vi "MotorParam_mm_to_ct.vi"(10 "Motor Parameters (Natural Units)":T1={"velocity mm/s"=[10.0, 10.0, 10.0, 20.0], "accel mm/s^2"=[50.0, 50.0, 50.0, 200.0]}, 11 "Counts / mm":i32[](array[numeric])=[1000, 1000, 1000, 1000]) -> (3 "Motoar Parameters (counts)":cluster{dbl[], dbl[]})   [LabVIEW 2022 SP3]
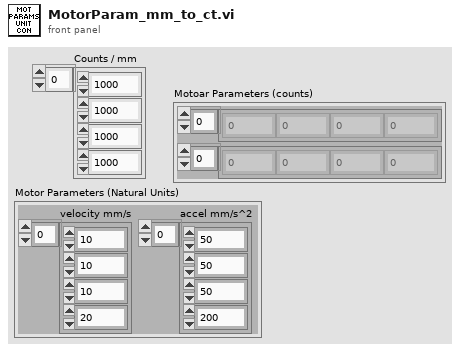
[diagram p1: front panel]
types:
  T1 = cluster{"velocity mm/s":dbl[], "accel mm/s^2":dbl[]}
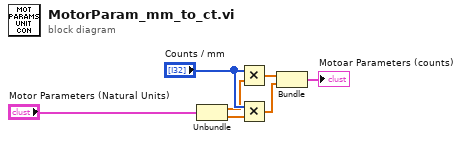
[diagram p0: block diagram]
diagram:
  n1 = Unbundle("Motor Parameters (Natural Units)") -> ("velocity mm/s"=w5:dbl[], "accel mm/s^2"=w1:dbl[])
  n2 = Multiply(x="Counts / mm", y=w5) -> (x*y=w3:dbl[])
  n3 = Multiply(x="Counts / mm", y=w1) -> (x*y=w4:dbl[])
  n4 = Bundle(w3, w4) -> (→"Motoar Parameters (counts)":cluster{dbl[], dbl[]})  [unwired: 1 in]
